vi "GetConfigFilesPath.vi"(8 "error in (no error)":errorcluster, 11 "Model in":refnum<class "Model.lvclass">) -> (0 "error out":errorcluster, 2 "ConfigFilesPath":T1, 3 "Model out":refnum<class "Model.lvclass">)   [LabVIEW 2016, in "Model.lvclass"]
uses:
  Model.lvclass
  Typedefs/ActuatorLocationPath.ctl
  Model.lvclass/Model.ctl
  Typedefs/M1M3SupportEUI_TypeDefs.lvlib
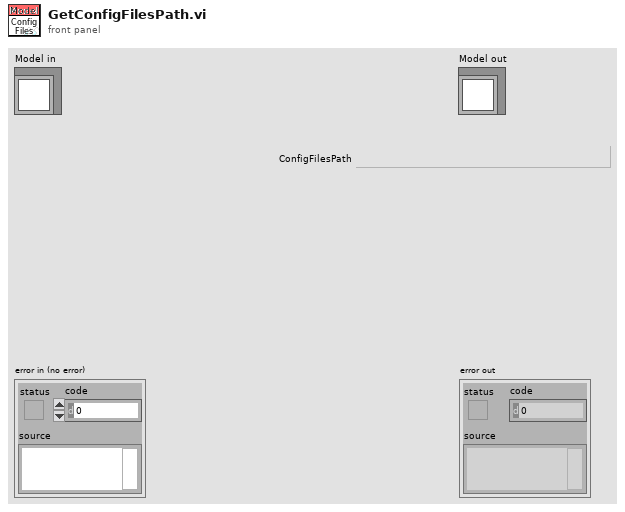
[diagram p1: front panel]
types:
  T1 = typedef "M1M3SupportEUI_TypeDefs.lvlib/ActuatorLocationPath.ctl" = path
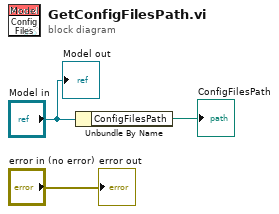
[diagram p0: block diagram]
diagram:
  n1 = Unbundle By Name("Model in") -> ("ConfigFilesPath"=→"ConfigFilesPath":T1)
  "error out" <- "error in (no error)"
  "Model out" <- "Model in"
